vi "_ObtainPrefixQueue.vi"(5 "PrefixQueue Type":refnum<class "PrefixQueue.lvclass">, 7 "Max Queue Size (-1, Unlimited)":i32=-1, 8 "error in (no error)":errorcluster, 10 "Create If Not Found? (T)":bool=TRUE, 11 "Queue Name":string) -> (0 "error out":errorcluster, 1 "Created New?":bool, 3 "PrefixQueue out":refnum<class "PrefixQueue.lvclass">)   [LabVIEW 2017, in "LapDog.Messaging.v3.PrefixQueue.lvlib" / "PrefixQueue.lvclass"]
doc: "Creates a PrefixQueue object. \n\nChild classes should use this method in their creator method, passing a child class object in on the PrefixQueue Type terminal."
uses:
  PrefixQueue.lvclass
  C:/git/LapDog.Messaging/src/LapDog.Messaging/MessageQueue/MessageQueue.lvclass
  PrefixQueue.lvclass/PrefixQueue.ctl
  LapDog.Messaging/MessageQueue/MessageQueue.lvclass
panel:
  in  "Message Name Prefix":string
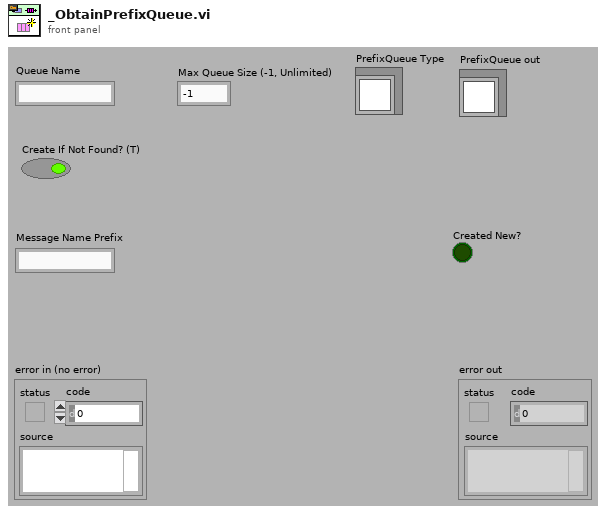
[diagram p1: front panel]
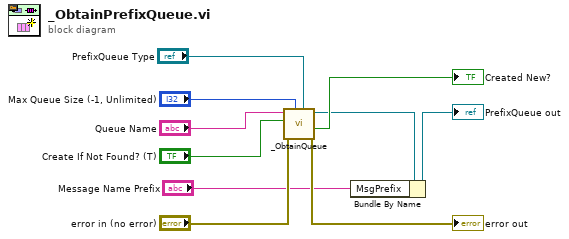
[diagram p0: block diagram]
diagram:
  n1 = call "_ObtainQueue.vi"("MessageQueue Type"="PrefixQueue Type", "Max Queue Size (-1, unlimited)"="Max Queue Size (-1, Unlimited)", "error in (no error)"="error in (no error)", "Create if Not Found? (T)"="Create If Not Found? (T)", "Queue Name"="Queue Name") -> ("error out"=→"error out":errorcluster, "Created New?"=→"Created New?":bool, "MessageQueue out"=w4:refnum<class "PrefixQueue.lvclass">)  [unwired: 4 in]
  n2 = Bundle By Name(cluster=w4, "MsgPrefix"="Message Name Prefix") -> (→"PrefixQueue out":refnum<class "PrefixQueue.lvclass">)
